vi "UpdateConfigCtls.vi"(6 "Units":refnum<vi>, 8 "error in (no error)":errorcluster, 9 "Type":refnum<vi>, 10 "Selected Channels":T1=[0], 11 "9212 in":refnum<class "9212.lvclass">) -> (0 "error out":errorcluster, 3 "9212 out":refnum<class "9212.lvclass">)   [LabVIEW 2019, in "Modules.lvlib" / "9212.lvclass"]
uses:
  9212.lvclass
  Channels Listbox.ctl
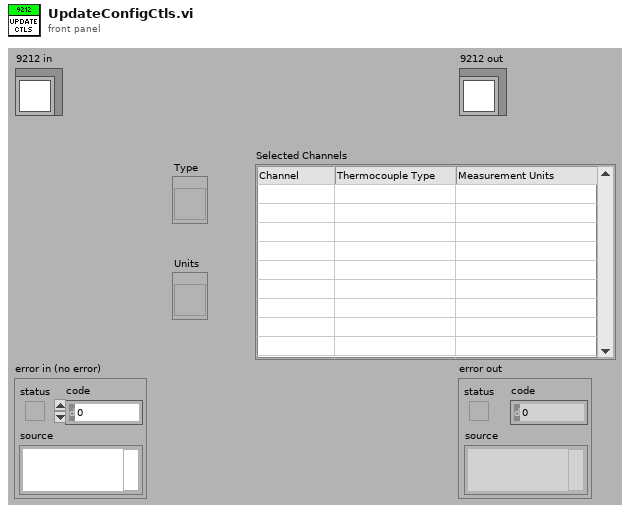
[diagram p1: front panel]
types:
  T1 = typedef "Modules.lvlib/9212.lvclass/Channels Listbox.ctl" = i32[]
  T2 = typedef "Modules.lvlib/9212.lvclass/Measurement Units.ctl" = u8
  T3 = typedef "Modules.lvlib/9212.lvclass/Thermocouple Type.ctl" = u8
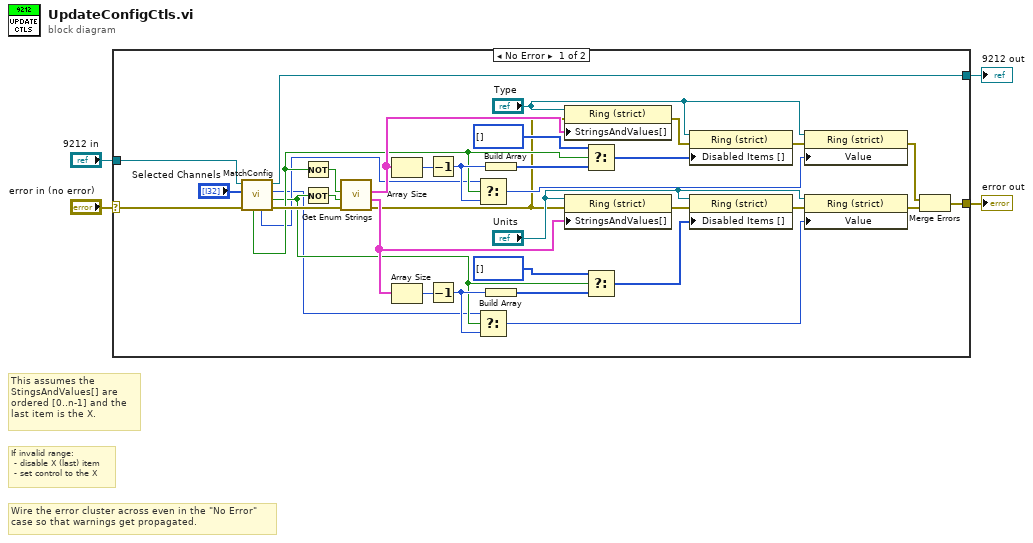
[diagram p0: block diagram]
diagram:
  # "Wire the error cluster across even in the \"No Error\"\ncase so that warnings get propagated."
  # "This assumes the StingsAndValues[] are ordered [0..n-1] and the last item is the X."
  # "If invalid range:\n - disable X (last) item\n - set control to the X"
  n1 = case shown="No Error" "error in (no error)" {
    selector: "error in (no error)" -> [w14 w41]
    tunnel: [w5 w41] -> w3
    tunnel: [w16 w40] -> w1
    tunnel: "9212 in" -> [w17 w40]
    frame No Error {
      n2 = call "MatchConfig.vi"("error in (no error)"=w14, "Selected Channels"="Selected Channels", "9212 in"=w17) -> ("error out"=w13:errorcluster, "All same DegreeRange?"=w11:bool, "DegreeRange value"=w9:T2, "9212 out"=w16:refnum<class "9212.lvclass">, "TCoupleType value"=w10:T3, "All same TCoupleType?"=w12:bool)  [unwired: 3 in]
      n3 = Not(x=w12) -> (.not. x?=w19:bool)
      n4 = Not(x=w11) -> (.not. x?=w18:bool)
      n5 = call "Get Enum Strings.vi"("error in (no error)"=w13, "Units"=w18, "Type"=w19) -> ("error out"=w8:errorcluster, "Units"=w20:cluster{"String":string, "Value":u16}[], "Type"=w21:cluster{"String":string, "Value":u16}[])  [unwired: 6 in]
      n6 = Array Size(array=w21) -> (size(s)=w29:i32)
      n7 = Array Size(array=w20) -> (size(s)=w26:i32)
      n8 = Decrement(x=w29) -> (x-1=w28:i32)
      n9 = Decrement(x=w26) -> (x-1=w27:i32)
      n10 = Select(t=w10, s=w12, f=w28) -> (s? t:f=w39:i32)
      n11 = Select(t=w9, s=w11, f=w27) -> (s? t:f=w33:i32)
      n12 = Build Array(w28) -> (w30:i32[])
      n13 = Build Array(w27) -> (w25:i32[])
      n14 = property on="Property Node" class="Ring (strict)"(reference="Type", error in=w8, "StringsAndValues[]"=w21) -> (error out=w37:errorcluster)  [unwired: 1 out]
      n15 = property on="Property Node" class="Ring (strict)"(reference="Units", error in=w8, "StringsAndValues[]"=w20) -> (error out=w34:errorcluster)  [unwired: 1 out]
      n16 = Select(t=i32[] [], s=w12, f=w30) -> (s? t:f=w38:i32[])
      n17 = Select(t=i32[] [], s=w11, f=w25) -> (s? t:f=w32:i32[])
      n18 = property on="Property Node" class="Ring (strict)"(reference="Type", error in=w37, "Disabled Items []"=w38) -> (error out=w36:errorcluster)  [unwired: 1 out]
      n19 = property on="Property Node" class="Ring (strict)"(reference="Units", error in=w34, "Disabled Items []"=w32) -> (error out=w35:errorcluster)  [unwired: 1 out]
      n20 = property on="Property Node" class="Ring (strict)"(reference="Type", error in=w36, "Value"=w39) -> (error out=w7:errorcluster)  [unwired: 1 out]
      n21 = property on="Property Node" class="Ring (strict)"(reference="Units", error in=w35, "Value"=w33) -> (error out=w6:errorcluster)  [unwired: 1 out]
      n22 = Merge Errors(w7, w6) -> (w5:errorcluster)
    }
    frame Error {
    }
  }
  "error out" <- w3
  "9212 out" <- w1
